vi "ESP301 StopMot.vi"(5 "Axe Inv":bool, 6 "Input Units":i8(ring) items=["mm", "ps"], 7 "ESP301Ref":T1, 8 "error in":errorcluster, 9 "Axis":i8(ring)=1 items=["Axis 1"=1, "Axis 2"=2, "Axis 3"=3], 11 "VISA Rsrc":refnum<visa-resource-name>="GPIB0::7::INSTR") -> (0 "error out":errorcluster, 2 "Pos Out":dbl=0.5)   [LabVIEW 2019]
uses:
  <userlib>/ESP300/ESP300 GotoState.ctl
  <userlib>/GenProg/WritebyRefNum.vi
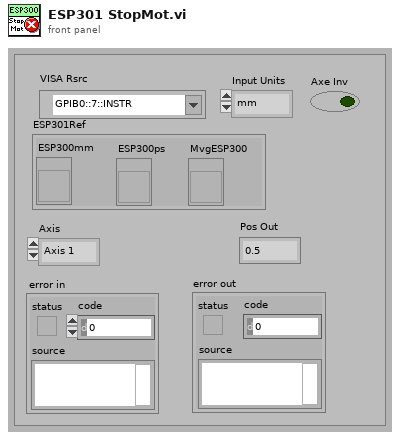
[diagram p1: front panel]
types:
  T1 = cluster{"ESP300mm":refnum<vi>, "ESP300ps":refnum<vi>, "MvgESP300":refnum<vi>}
  T2 = typedef "ESP300 GotoState.ctl" = enum16{"send command", "read position", "check status", "end"}
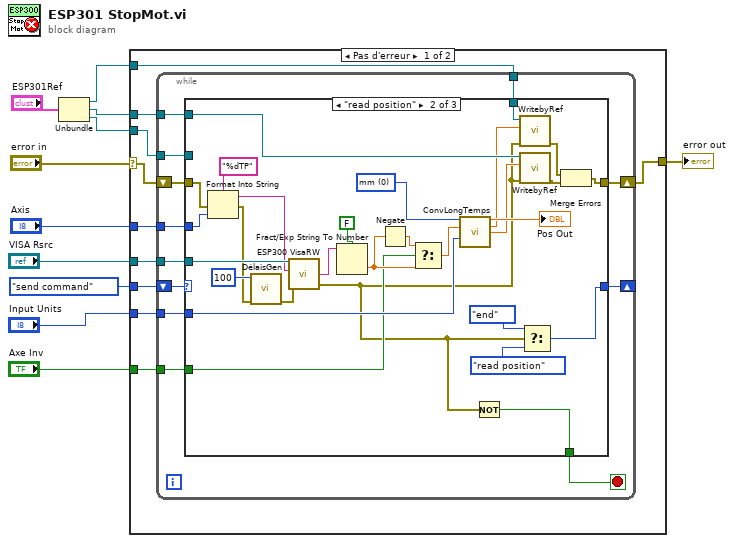
[diagram p0: block diagram]
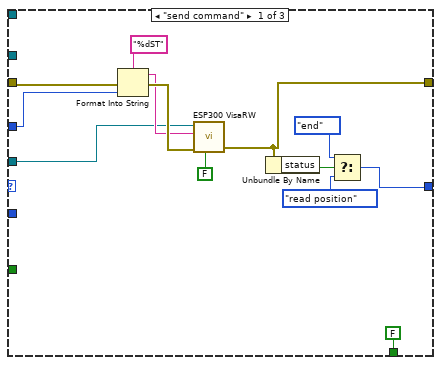
[diagram p2: hidden frame]
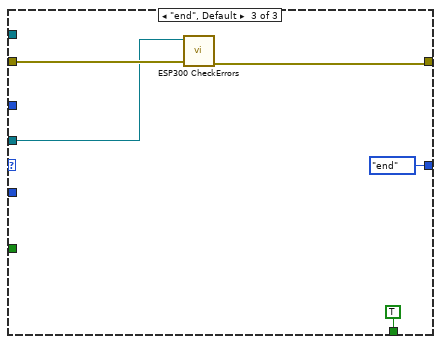
[diagram p3: hidden frame]
diagram:
  n1 = Unbundle("ESP301Ref") -> ("ESP300mm"=w2:refnum<vi>, "ESP300ps"=w4:refnum<vi>, "MvgESP300"=w3:refnum<vi>)
  n2 = case shown="Pas d'erreur" "error in" {
    selector: "error in" -> [w19 w81]
    tunnel: "Axis" -> [w21 _]
    tunnel: [w18 w81] -> w9
    tunnel: ESP300_GotoState."send command" ("Énum") -> [w20 _]
    tunnel: "VISA Rsrc" -> [w17 _]
    tunnel: w3 -> [w16 _]
    tunnel: "Input Units" -> [w15 _]
    tunnel: w2 -> [w14 _]
    tunnel: w4 -> [w13 _]
    tunnel: "Axe Inv" -> [w12 _]
    frame No Error {
      n3 = while {
        tunnel: w21 -> [w33]
        shift-right: [w29] -> w18
        shift-left: w19 -> [w31]
        tunnel: w17 -> [w30]
        shift-right: [w27] -> _
        shift-left: w20 -> [w32]
        tunnel: w16 -> [w26]
        tunnel: w15 -> [w25]
        tunnel: w14 -> [w24]
        tunnel: w13 -> [w23]
        tunnel: w12 -> [w22]
        stop <- w28 stop-if-true
        n4 = case shown="\"read position\"" w32 {
          tunnel: w33 -> [w35 w73 _]
          tunnel: w31 -> [w39 w72 w78]
          tunnel: w30 -> [w38 w75 w76]
          tunnel: [w36 w61 w77] -> w29
          tunnel: [FALSE w47 TRUE] -> w28
          tunnel: [w37 w66 ESP300_GotoState."end" ("Énum")] -> w27
          tunnel: w26 -> [_ _ _]
          tunnel: w25 -> [_ w53 _]
          tunnel: w24 -> [_ w59 _]
          tunnel: w23 -> [_ w58 _]
          tunnel: w22 -> [_ w49 _]
          frame "send command" {
            n5 = Format Into String(format string="%dST", error in=w39, w35) -> (resulting string=w44:string, error out=w45:errorcluster)  [unwired: 1 in]
            n6 = call <userlib>:"ESP300 VisaRW.vi"("Lecture?(T)"=FALSE, "error in (no error)"=w45, "ChaineCom"=w44, "VISA Rsrc"=w38) -> ("error out"=w36:errorcluster)  [unwired: 3 in, 3 out]
            n7 = Unbundle By Name(w36) -> ("status"=w42:bool)
            n8 = Select(t=ESP300_GotoState."end" ("Énum"), s=w42, f=ESP300_GotoState."read position" ("Énum")) -> (s? t:f=w37:T2)
          }
          frame "read position" {
            w57 = i8 0 items=["mm", "ps"] ("Input Units")
            n9 = Format Into String(format string="%dTP", error in=w72, w73) -> (resulting string=w71:string, error out=w63:errorcluster)  [unwired: 1 in]
            n10 = call "DélaisGen.vi"("error in (no error)"=w63, "ms To Wait"=u32 100 ("milliseconds to wait")) -> ("error out"=w64:errorcluster)  [unwired: 9 in]
            n11 = call <userlib>:"ESP300 VisaRW.vi"("error in (no error)"=w64, "ChaineCom"=w71, "VISA Rsrc"=w75) -> ("error out"=w48:errorcluster, "ChaineRep"=w70:string)  [unwired: 4 in, 2 out]
            n12 = Fract/Exp String To Number(use system decimal point (T)=FALSE ("utiliser le séparateur décimal du système (V)"), string=w70) -> (number=w51:dbl)  [unwired: 2 in, 1 out]
            n13 = Negate(x=w51) -> (-x=w52:dbl)
            n14 = Select(t=w52, s=w49, f=w51) -> (s? t:f=w50:dbl)
            n15 = call <userlib>:"ConvLongTemps.vi"("Input Units"=w57, "Units Input"=w50, "Output Units"=w53) -> ("Units Output"=→"Pos Out":dbl, "Units mm"=w55:dbl, "Units ps"=w54:dbl)  [unwired: 9 in, 1 out]
            n16 = Not(x=w48) -> (.not. x?=w47:bool)
            n17 = call-poly <userlib>:"WritebyRef.vi"("error in"=w48, "Valeur"=w55, "Control Ref"=w59) -> ("error out"=w60:errorcluster)  [unwired: 8 in]
            n18 = call-poly <userlib>:"WritebyRef.vi"("error in"=w48, "Valeur"=w54, "Control Ref"=w58) -> ("error out"=w62:errorcluster)  [unwired: 8 in]
            n19 = Select(t=ESP300_GotoState."end" ("Énum"), s=w48, f=ESP300_GotoState."read position" ("Énum")) -> (s? t:f=w66:T2)
            n20 = Merge Errors(w60, w62) -> (w61:errorcluster)
          }
          frame "end", Default {
            n21 = call <userlib>:"ESP300 CheckErrors.vi"("error in (no error)"=w78, "Ressource VISA In"=w76) -> ("error out"=w77:errorcluster)  [unwired: 4 in, 3 out]
          }
        }
      }
    }
    frame Error {
    }
  }
  "error out" <- w9
